vi "Update Tree.vi"(7 "Filter Fails?":bool, 8 "error in (no error)":errorcluster, 9 "Test Tree":refnum<vi>, 10 "Result Model":refnum<class "Result Model.lvclass">) -> (0 "error out":errorcluster)   [LabVIEW 2020, in "Execution UI V2.lvclass"]
uses:
  Execution UI V2.lvclass
  Result Model/Result Model.lvclass
  Execution UI V2.lvclass/Execution UI V2.ctl
  Result Model/Tree Item Filter.ctl
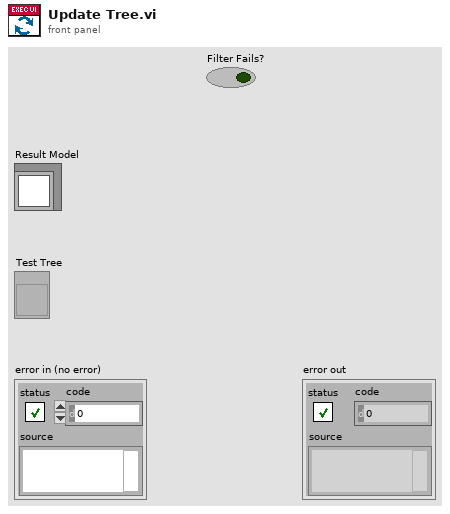
[diagram p1: front panel]
types:
  T1 = typedef "Result Model.lvclass/Tree Item Filter.ctl" = enum16{"All", "Only Fails"}
  T2 = cluster{"Left Cell String":string, "Child Text":string[], "Child Tag":string, "Item Indent":i32, "Child Only?":bool, "Glyph Index":i32}[]
  T3 = typedef "LVNodeAndColumnTypeDef.ctl" = cluster{"Node":string, "Column":i32}
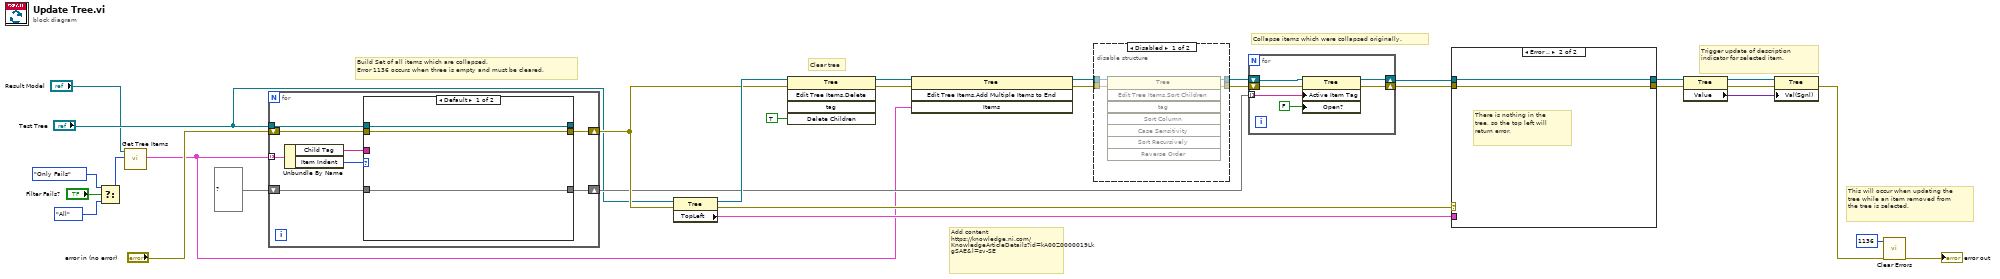
[diagram p0: block diagram]
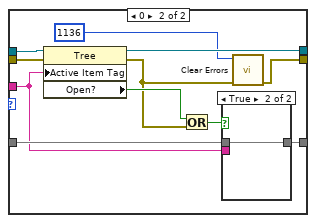
[diagram p3: hidden frame]
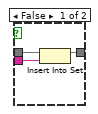
[diagram p4: hidden frame]
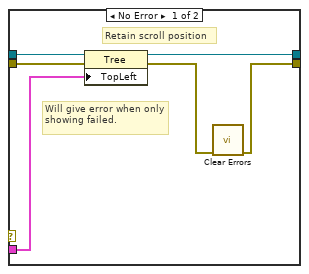
[diagram p5: hidden frame]
diagram:
  # "Collapse items which were collapsed originally."
  # "Build Set of all items which are collapsed.\nError 1136 occurs when three is empty and must be cleared."
  # "This will occur when updating the tree while an item removed from the tree is selected."
  # "Trigger update of description indicator for selected item."
  # "Add content\nhttps://knowledge.ni.com/KnowledgeArticleDetails?id=kA00Z0000019LkgSAE&l=sv-SE"
  # "Clear tree"
  n1 = Select(t=Tree_Item_Filter."Only Fails" ("Filter"), s="Filter Fails?", f=Tree_Item_Filter."All" ("Filter")) -> (s? t:f=w2:T1)
  n2 = call "Get Tree Items.vi"("Filter"=w2, "Result Model In"="Result Model") -> ("Tree Items"=w7:T2)  [unwired: 9 in]
  n3 = for {
    tunnel: w7 -> [w39] mode=indexing
    shift-right: [w33] -> w18
    shift-left: "error in (no error)" -> [w34]
    shift-right: [w36] -> w16
    shift-left: set{string} {} ("set") -> [w37]
    tunnel: "Test Tree" -> [w38]
    n4 = Unbundle By Name(w39) -> ("Child Tag"=w35:string, "Item Indent"=w32:i32)
    n5 = case shown="Default" w32 {
      tunnel: w38 -> [w41 w53]
      tunnel: [w41 w52] -> _
      tunnel: w37 -> [w42 w51]
      tunnel: [w42 w50] -> w36
      tunnel: w35 -> [_ w49]
      tunnel: w34 -> [w40 w47]
      tunnel: [w40 w46] -> w33
      frame Default {
      }
      frame 0 {
        n6 = property class="Tree"(reference=w53, error in=w47, "Active Item Tag"=w49) -> (reference out=w52:refnum<vi>, error out=w43:errorcluster, "Open?"=w48:bool)
        n7 = Or(x=w48, y=w43) -> (x .or. y?=w44:bool)
        n8 = case shown="True" w44 {
          tunnel: w51 -> [w56 w57]
          tunnel: [w55 w57] -> w50
          tunnel: w49 -> [w54 _]
          frame False {
            n9 = Insert Into Set(10:w54, 11:w56) -> (3:w55:set{string})  [unwired: 1 out]
          }
          frame True {
          }
        }
        n10 = call <vilib>:"Clear Errors.vi"("error in (no error)"=w43, "specific error code to clear (0: all)"=1136) -> ("error out"=w46:errorcluster)  [unwired: 4 in, 1 out]
      }
    }
  }
  n11 = property on="Property Node" class="Tree"(reference="Test Tree", error in=w18) -> (reference out=w28:refnum<vi>, error out=w27:errorcluster, "TopLeft"=w26:T3)
  n12 = invoke on="Invoke Node" class="Tree" method="Edit Tree Items.Delete"(reference=w28, error in=w18, "Delete Children"=TRUE ("Delete Children?")) -> (reference out=w30:refnum<vi>, error out=w29:errorcluster)  [unwired: 2 in, 3 out]
  n13 = invoke class="Tree" method="Edit Tree Items.Add Multiple Items to End"(reference=w30, error in=w29, "Items"=w7) -> (reference out=w13:refnum<vi>, error out=w9:errorcluster)  [unwired: 1 in, 2 out]
  n14 = disable-structure shown="Disabled" {
    disable-tunnel: w13 -> [w61 w63]
    disable-tunnel: [w60 w63] -> w10
    disable-tunnel: w9 -> [w59 w62]
    disable-tunnel: [w58 w62] -> w8
    frame Disabled {
      n15 = invoke class="Tree" method="Edit Tree Items.Sort Children"(reference=w61, error in=w59) -> (reference out=w60:refnum<vi>, error out=w58:errorcluster)  [unwired: 6 in, 6 out]
    }
    frame Enabled {
    }
  }
  n16 = for {
    shift-right: [w68] -> w12
    shift-left: w10 -> [w69]
    shift-right: [w67] -> w11
    shift-left: w8 -> [w66]
    tunnel: w16 -> [w65] mode=indexing
    n17 = property class="Tree"(reference=w69, error in=w66, "Active Item Tag"=w65, "Open?"=FALSE ("Active Item:Open?")) -> (reference out=w68:refnum<vi>, error out=w67:errorcluster)
  }
  n18 = case shown="Error .." w27 {
    tunnel: w12 -> [w75 w77]
    tunnel: [w74 w77] -> w15
    tunnel: w11 -> [w73 w76]
    tunnel: [w70 w76] -> w14
    tunnel: w26 -> [w71 _]
    frame No Error {
      # "Will give error when only showing failed."
      # "Retain scroll position"
      n19 = property on="Property Node" class="Tree"(reference=w75, error in=w73, "TopLeft"=w71) -> (reference out=w74:refnum<vi>, error out=w72:errorcluster)
      n20 = call <vilib>:"Clear Errors.vi"("error in (no error)"=w72) -> ("error out"=w70:errorcluster)  [unwired: 5 in, 1 out]
    }
    frame Error {
      # "There is nothing in the tree, so the top left will return error."
    }
  }
  n21 = property on="Property Node" class="Tree"(reference=w15, error in=w14) -> (reference out=w25:refnum<vi>, error out=w24:errorcluster, "Value"=w22:variant)
  n22 = property on="Property Node" class="Tree"(reference=w25, error in=w24, "Val(Sgnl)"=w22) -> (error out=w23:errorcluster)  [unwired: 1 out]
  n23 = call <vilib>:"Clear Errors.vi"("error in (no error)"=w23, "specific error code to clear (0: all)"=1136) -> ("error out"=→"error out":errorcluster)  [unwired: 4 in, 1 out]
